vi "Set Task List.vi"(8 "error in (no error)":errorcluster, 10 "Task List":refnum<class "Task.lvclass">[](array[class]), 11 "Task Setting Editor in":refnum<class "Task Setting Editor.lvclass">) -> (0 "error out":errorcluster, 3 "Task Setting Editor out":refnum<class "Task Setting Editor.lvclass">)   [LabVIEW 2017, in "Task Setting Editor.lvlib" / "Task Setting Editor.lvclass"]
uses:
  Task Setting Editor.lvclass
  Classes/Task Interface/Task/Task.lvclass
  Task Setting Editor.lvclass/Task Setting Editor.ctl
  Classes/Task Interface/Task/Task.lvclass/Task.ctl
  Classes/Task Interface/Task/Get Name.vi
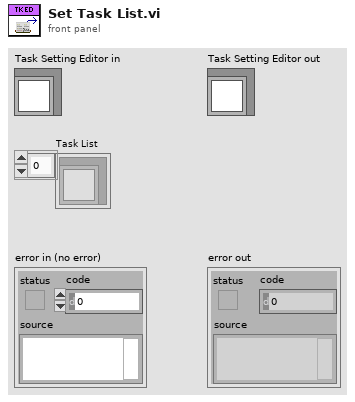
[diagram p1: front panel]
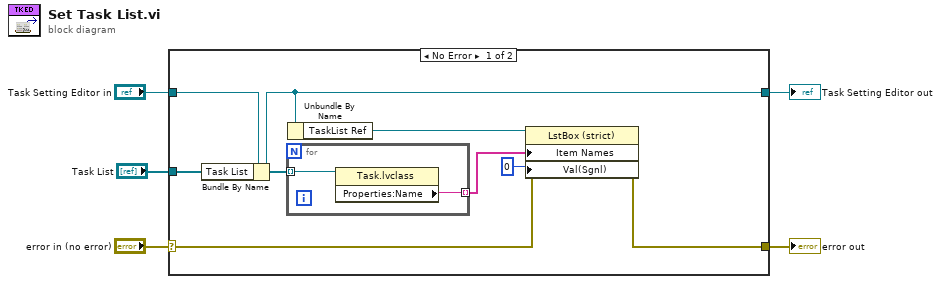
[diagram p0: block diagram]
diagram:
  n1 = case shown="No Error" "error in (no error)" {
    selector: "error in (no error)" -> [w11 w17]
    tunnel: [w10 w17] -> w4
    tunnel: [w7 w16] -> w2
    tunnel: "Task Setting Editor in" -> [w8 w16]
    tunnel: "Task List" -> [w6 _]
    frame No Error {
      n2 = Bundle By Name(cluster=w8, "Task List"=w6) -> (w7:refnum<class "Task Setting Editor.lvclass">)
      n3 = for {
        tunnel: w6 -> [w14] mode=indexing
        tunnel: [w15] -> w12 mode=indexing
        n4 = property class="Task.lvclass"(reference=w14) -> ("Properties:Name"=w15:string)  [unwired: 1 in, 2 out]
      }
      n5 = Unbundle By Name(w7) -> ("TaskList Ref"=w13:refnum<vi>)
      n6 = property class="LstBox (strict)"(reference=w13, error in=w11, "Item Names"=w12, "Val(Sgnl)"=0 ("Value (Signaling)")) -> (error out=w10:errorcluster)  [unwired: 1 out]
    }
    frame Error {
    }
  }
  "error out" <- w4
  "Task Setting Editor out" <- w2
